vi "LoadLegacyArmPressure.vi"(8 "error in (no error)":errorcluster, 11 "File path":path) -> (0 "error out":errorcluster, 2 "Left":T1(array[cluster]), 3 "Right":T1(array[cluster]))   [LabVIEW 2013, in "main.lvlib"]
uses:
  main.lvlib
  Globals/DataPathGlobalVariable.vi
  <userlib>/_OpenG.lib/file/file.llb/File Exists - Scalar__ogtk.vi
  <vilib>/Utility/file.llb/Read From Spreadsheet File (DBL).vi
panel:
  out "all rows":dbl[][](array[numeric]) format="%0.3f"
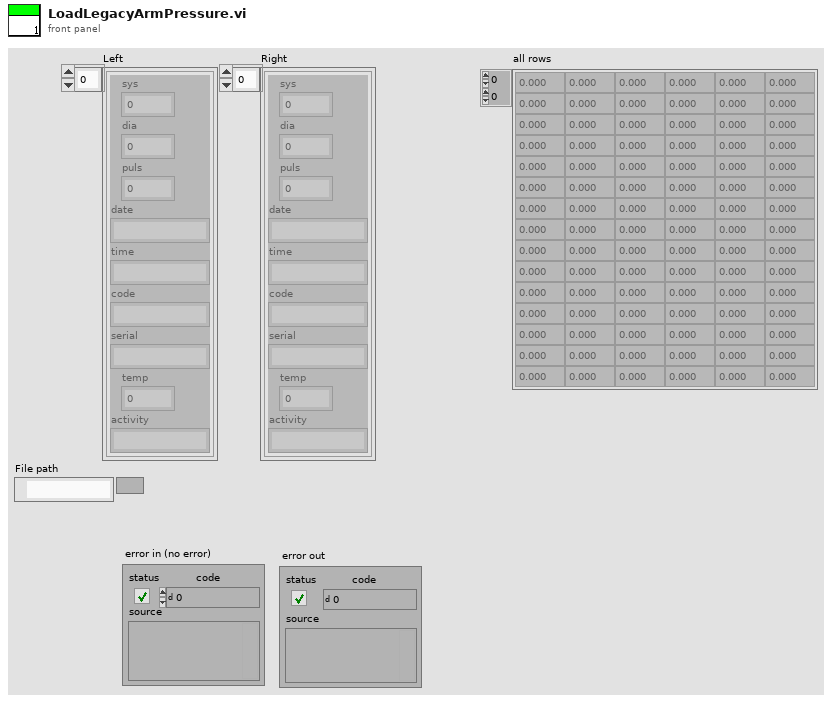
[diagram p1: front panel]
types:
  T1 = cluster{"sys":dbl, "dia":dbl, "puls":dbl, "date":string, "time":string, "code":string, "serial":string, "temp":dbl, "activity":string}[]
  T2 = cluster{"sys":dbl, "dia":dbl, "puls":dbl, "date":string, "time":string, "code":string, "serial":string, "temp":dbl, "activity":string}
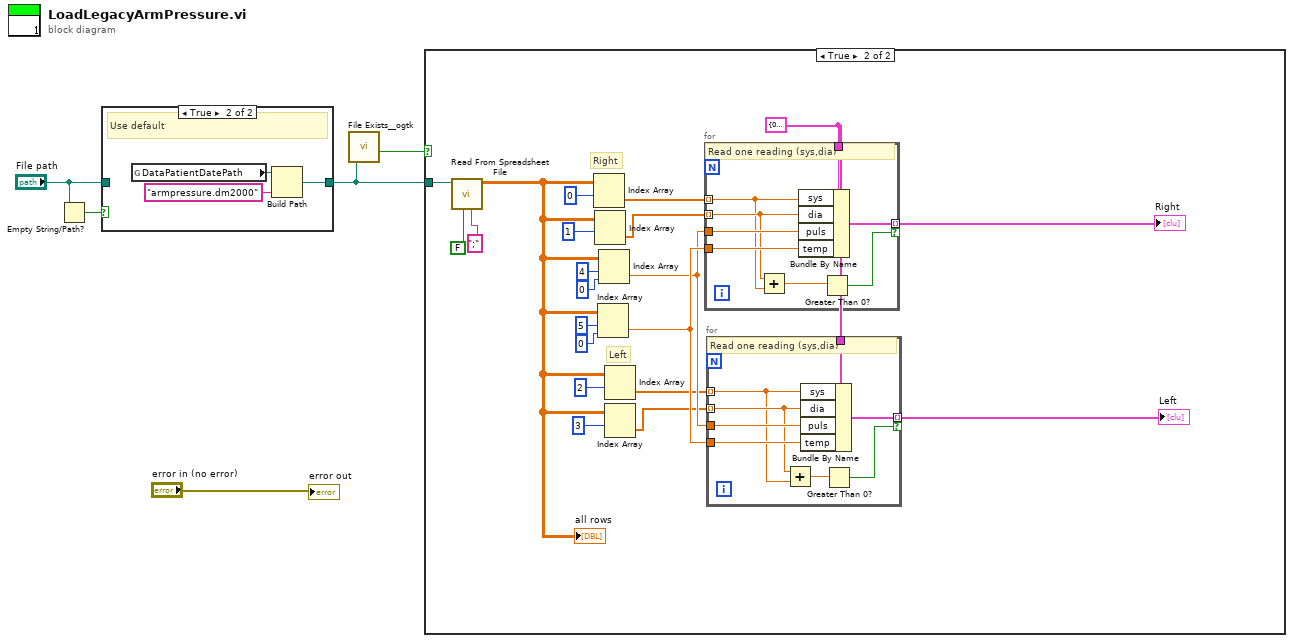
[diagram p0: block diagram]
diagram:
  n1 = Empty String/Path?(string/path="File path") -> (empty?=w3:bool)
  n2 = case shown="True" w3 {
    tunnel: [w6 w7] -> w4
    tunnel: "File path" -> [w6 _]
    frame False {
    }
    frame True {
      # "Use default"
      n3 = global read "DataPathGlobalVariable.vi" "DataPatientDatePath"() -> (w9:path)
      n4 = Build Path(base path=w9, name or relative path="armpressure.dm2000") -> (appended path=w7:path)
    }
  }
  n5 = call-poly <userlib>:"File Exists__ogtk.vi"("file path"=w4) -> ("exists"=w5:bool)  [unwired: 6 in, 1 out]
  n6 = case shown="True" w5 {
    tunnel: w4 -> [_ w28]
    frame False {
    }
    frame True {
      w23 = T2 {"sys"=0.0, "dia"=0.0, "puls"=0.0, "date"="", "time"="", "code"="", "serial"="", "temp"=0.0, "activity"=""} ("data")
      # "Right"
      # "Left"
      n7 = call-poly <vilib>:"Read From Spreadsheet File.vi"("delimiter (\\t)"=";" ("delimiter (\\t)"), "transpose (no:F)"=FALSE, "file path (dialog if empty)"=w28) -> ("all rows"=w18:dbl[][])  [unwired: 4 in, 4 out]
      "all rows" <- w18
      n8 = Index Array(array=w18, index (row)=0) -> (element=w20:dbl[])  [unwired: 1 in]
      n9 = Index Array(array=w18, index (row)=1) -> (element=w19:dbl[])  [unwired: 1 in]
      n10 = Index Array(array=w18, index (row)=5 ("index"), index (col)=0 ("length")) -> (element=w22:dbl)
      n11 = Index Array(array=w18, index (row)=4 ("index"), index (col)=0 ("length")) -> (element=w21:dbl)
      n12 = Index Array(array=w18, index (row)=2) -> (element=w17:dbl[])  [unwired: 1 in]
      n13 = Index Array(array=w18, index (row)=3) -> (element=w16:dbl[])  [unwired: 1 in]
      n14 = for {
        tunnel: w23 -> [w46]
        tunnel: [w45] -> w11 mode=indexing if=w44
        tunnel: w21 -> [w43]
        tunnel: w22 -> [w42]
        tunnel: w20 -> [w39] mode=indexing
        tunnel: w19 -> [w40] mode=indexing
        # "Read one reading (sys,dia)"
        n15 = Add(x=w40, y=w39) -> (x+y=w41:dbl)
        n16 = Bundle By Name(cluster=w46, "sys"=w39, "dia"=w40, "puls"=w43, "temp"=w42) -> (w45:T2)
        n17 = Greater Than 0?(x=w41) -> (x > 0?=w44:bool)
      }
      "Right" <- w11
      n18 = for {
        tunnel: w23 -> [w38]
        tunnel: [w37] -> w10 mode=indexing if=w36
        tunnel: w21 -> [w35]
        tunnel: w22 -> [w34]
        tunnel: w17 -> [w32] mode=indexing
        tunnel: w16 -> [w33] mode=indexing
        # "Read one reading (sys,dia)"
        n19 = Add(x=w33, y=w32) -> (x+y=w31:dbl)
        n20 = Bundle By Name(cluster=w38, "sys"=w32, "dia"=w33, "puls"=w35, "temp"=w34) -> (w37:T2)
        n21 = Greater Than 0?(x=w31) -> (x > 0?=w36:bool)
      }
      "Left" <- w10
    }
  }
  "error out" <- "error in (no error)"
